vi "NF LI56xx dvr Close.vi"(8 "error in (no error)":errorcluster caption="Error IN", 11 "VISA resource name":refnum<visa-resource-name>="GPIB0::2::INSTR") -> (0 "error out":errorcluster caption="Error OUT", 3 "VISA resource name out":refnum<visa-resource-name>)   [LabVIEW 2019]
doc: "close the interface of instrumet."
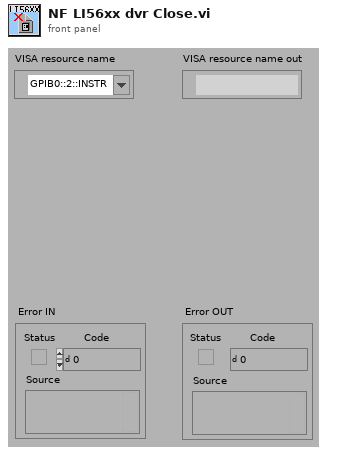
[diagram p1: front panel]
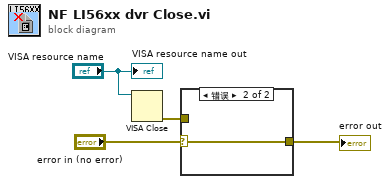
[diagram p0: block diagram]
diagram:
  n1 = VISA Close(VISA resource name="VISA resource name") -> (error out=w4:errorcluster)  [unwired: 1 in]
  n2 = case shown="错误" "error in (no error)" {
    selector: "error in (no error)" -> [_ w6]
    tunnel: [w5 w6] -> w2
    tunnel: w4 -> [w5 _]
    frame No Error {
    }
    frame Error {
    }
  }
  "error out" <- w2
  "VISA resource name out" <- "VISA resource name"
